vi "Timer Start.vi"(8 "error in (no error)":errorcluster, 11 "LV Server in":refnum<class "LV Server.lvclass">) -> (0 "error out":errorcluster, 3 "LV Server out":refnum<class "LV Server.lvclass">)   [LabVIEW 2020, in "LV Server.lvclass"]
uses:
  LV Server.lvclass
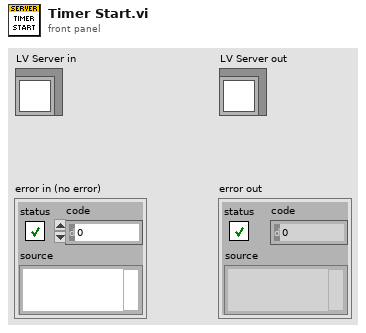
[diagram p1: front panel]
types:
  T1 = typedef "LV Server.lvclass/Timer Data.ctl" = cluster{"Start":dbl, "Accumulated":dbl, "Running":bool}
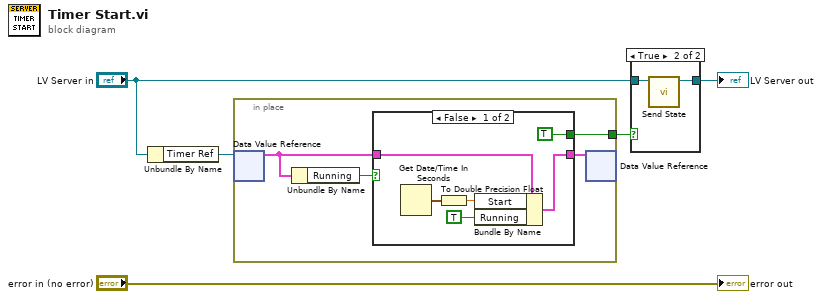
[diagram p0: block diagram]
diagram:
  n1 = Unbundle By Name("LV Server in") -> ("Timer Ref"=w4:refnum<data-value>)
  n2 = in-place {
    in-place-border: [w6] -> w3
    n3 = in-place-dvr #1(w4) -> (w8:T1)  [unwired: 1 out]
    n4 = Unbundle By Name(w8) -> ("Running"=w7:bool)
    n5 = case shown="False" w7 {
      tunnel: [w15 w16] -> w9
      tunnel: w8 -> [w11 w16]
      tunnel: [TRUE _] -> w6
      frame False {
        n6 = Get Date/Time In Seconds() -> (seconds since 1Jan1904=w13:timestamp)
        n7 = To Double Precision Float(number=w13) -> (double precision float=w12:dbl)
        n8 = Bundle By Name(cluster=w11, "Start"=w12, "Running"=TRUE) -> (w15:T1)
      }
      frame True {
      }
    }
    n9 = in-place-dvr #1(w9) -> ()  [unwired: 2 out]
  }
  n10 = case shown="True" w3 {
    tunnel: "LV Server in" -> [w17 w19]
    tunnel: [w17 w18] -> w1
    frame False {
    }
    frame True {
      n11 = call "Send State.vi"("LV Server in"=w19) -> ("LV Server out"=w18:refnum<class "LV Server.lvclass">)  [unwired: 9 in, 1 out]
    }
  }
  "LV Server out" <- w1
  "error out" <- "error in (no error)"
